vi "GetNextMatlabEvent.vi"(11 "ExperimentID":string) -> (1 "Numeric":dbl, 2 "String 2":string, 3 "String":string)   [LabVIEW 2017]
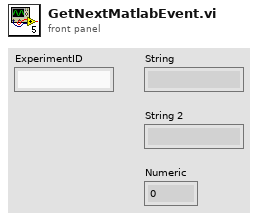
[diagram p1: front panel]
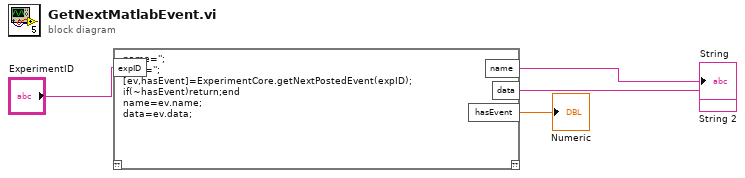
[diagram p0: block diagram]
diagram:
  n1 = script code="name='';\ndata='';\n[ev,hasEvent]=ExperimentCore.getNextPostedEvent(expID);\nif(~hasEvent)return;end\nname=ev.name;\ndata=ev.data;"("expID"="ExperimentID") -> ("name"=→"String":string, "data"=→"String 2":string, "hasEvent"=→"Numeric":dbl)  [unwired: 1 in, 1 out]
